vi "Home Filter Wheel.vi"(8 "error in (no error)":errorcluster, 10 "Motor":i32, 11 "FW Arduino Control in":refnum<class "FW Arduino Control.lvclass">) -> (0 "error out":errorcluster, 1 "Success":bool, 2 "Log":string, 3 "FW Arduino Control out":refnum<class "FW Arduino Control.lvclass">)   [LabVIEW 2021, in "FW Arduino Control.lvclass"]
uses:
  FW Arduino Control.lvclass
  C:/Development/prime/Prime-RIMAS/Filter Wheel/Filter Wheel Object/Filter Wheel.lvclass
  FW Arduino Control.lvclass/FW Arduino Control.ctl
  Filter Wheel Object/Filter Wheel.lvclass
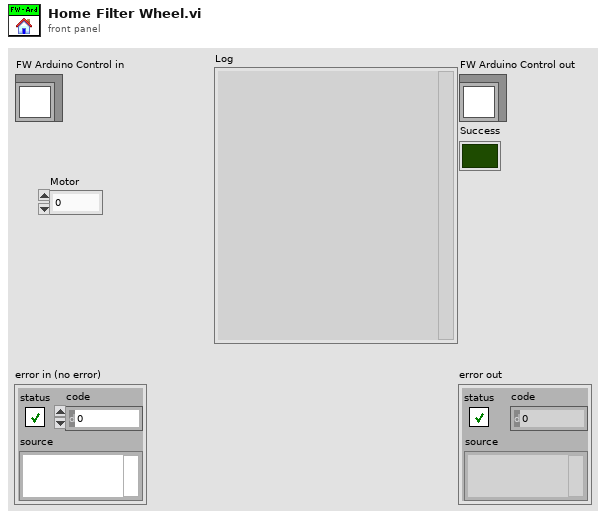
[diagram p1: front panel]
types:
  T1 = typedef "Filter Wheel Arduino Homing cluster.ctl" = cluster{"Direction (F: CW)":bool, "Speed":i32, "Accel":i32, "Min Distance":i32, "Short Leg":i32, "Error Cnts":i32}
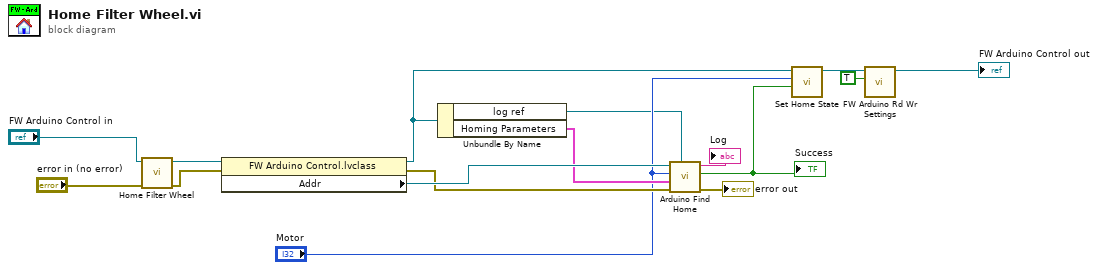
[diagram p0: block diagram]
diagram:
  n1 = call-parent "Home Filter Wheel.vi"("error in (no error)"="error in (no error)", "Filter Wheel in"="FW Arduino Control in") -> ("error out"=w13:errorcluster, "Filter Wheel out"=w14:refnum<class "FW Arduino Control.lvclass">)  [unwired: 6 in, 2 out]
  n2 = property class="FW Arduino Control.lvclass"(reference=w14, error in=w13) -> (reference out=w4:refnum<class "FW Arduino Control.lvclass">, error out=w11:errorcluster, "Addr"=w12:refnum<visa-resource-name>)
  n3 = Unbundle By Name(w4) -> ("log ref"=w5:refnum<file>, "Homing Parameters"=w9:T1)
  n4 = call "Arduino Find Home.vi"("log ref"=w5, "error in"=w11, "Homing Parameters"=w9, "Motor"="Motor", "Addr"=w12) -> ("error out"=→"error out":errorcluster, "Success"=w6:bool, "Log"=→"Log":string)  [unwired: 4 in]
  "Success" <- w6
  n5 = call "Set Home State.vi"("Home?"=w6, "Motor"="Motor", "Filter Wheel in"=w4) -> ("Filter Wheel out"=w3:refnum<class "FW Arduino Control.lvclass">)  [unwired: 7 in, 1 out]
  n6 = call "FW Arduino Rd Wr Settings.vi"("Write? (F:Read)"=TRUE, "Settings"=w3) -> ("Settings"=→"FW Arduino Control out":refnum<class "FW Arduino Control.lvclass">)  [unwired: 8 in, 1 out]
